vi "set_LSID.vi"(8 "error in (no error)":errorcluster, 10 "LSID":T1, 11 "GenericPlugin in":refnum<class "GenericComponent.lvclass">) -> (0 "error out":errorcluster, 3 "GenericPlugin out":refnum<class "GenericComponent.lvclass">)   [LabVIEW 2010, in "GenericComponent.lvclass"]
uses:
  GenericComponent.lvclass
  clusters/LSID_cluster.ctl
  GenericComponent.lvclass/GenericComponent.ctl
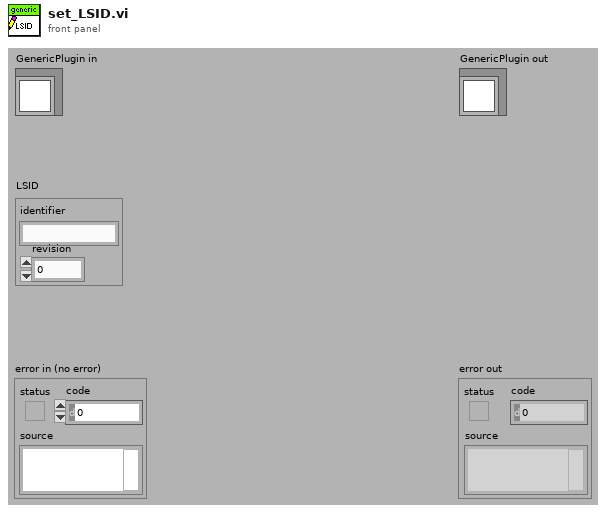
[diagram p1: front panel]
types:
  T1 = typedef "LSID_cluster.ctl" = cluster{"identifier":string, "revision":i32}
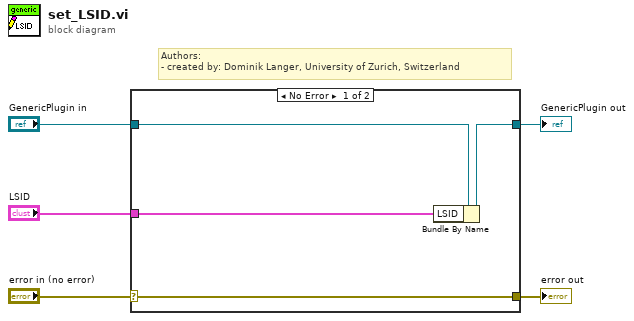
[diagram p0: block diagram]
diagram:
  # "Authors: \n- created by: Dominik Langer, University of Zurich, Switzerland"
  n1 = case shown="No Error" "error in (no error)" {
    selector: "error in (no error)" -> [w9 w10]
    tunnel: [w9 w10] -> w4
    tunnel: [w7 w11] -> w2
    tunnel: "GenericPlugin in" -> [w8 w11]
    tunnel: "LSID" -> [w6 _]
    frame No Error {
      n2 = Bundle By Name(cluster=w8, "LSID"=w6) -> (w7:refnum<class "GenericComponent.lvclass">)
    }
    frame Error {
    }
  }
  "error out" <- w4
  "GenericPlugin out" <- w2
